vi "Timer_Start.vi"(8 "error in (no error)":errorcluster caption="错误输入（无错误）", 11 "Timer 输入":refnum<class "Timer.lvclass">) -> (0 "error out":errorcluster caption="错误输出", 3 "Timer 输出":refnum<class "Timer.lvclass">)   [LabVIEW 2019, in "Timer.lvclass"]
uses:
  Timer.lvclass
  Timer_Core.vi
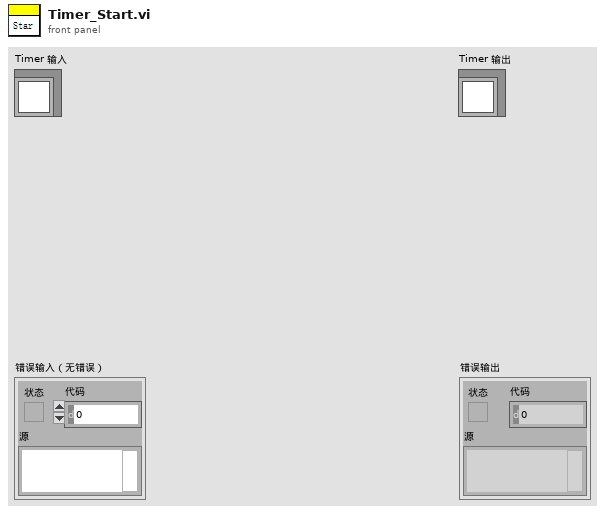
[diagram p1: front panel]
types:
  T1 = typedef "Timer.lvclass/Attribute.ctl" = cluster{"计时？":bool, "计时 (ms)":u32, "停止通知":refnum<notifier>}
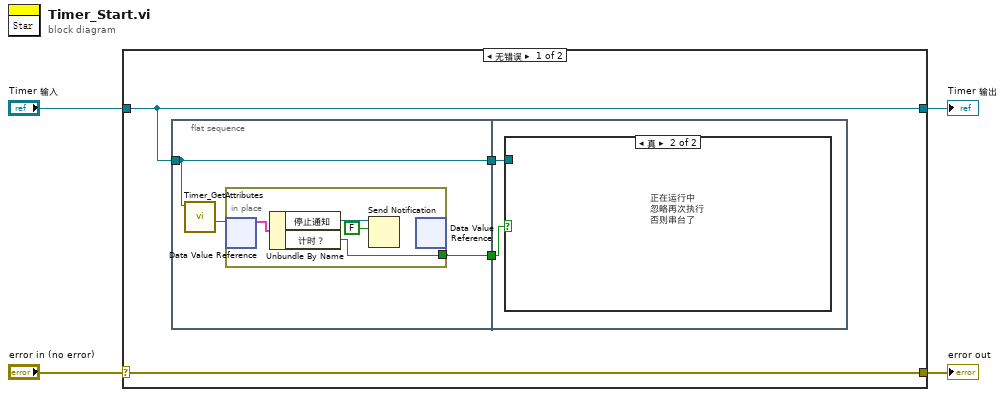
[diagram p0: block diagram]
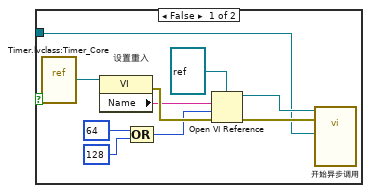
[diagram p2: hidden frame]
diagram:
  n1 = case shown="无错误" "error in (no error)" {
    selector: "error in (no error)" -> [w8 w29]
    tunnel: [w8 w29] -> w3
    tunnel: [w7 w28] -> w1
    tunnel: "Timer 输入" -> [w7 w28]
    frame No Error {
      n2 = flat-sequence {
        tunnel: w7 -> [w10]
        tunnel: [w10] -> w6
        tunnel: [w9] -> w5
        tunnel: w6 -> [w17]
        tunnel: w5 -> [w16]
        frame #0 {
          n3 = call "Timer_GetAttributes.vi"("Timer 输入"=w10) -> ("数据值引用"=w11:refnum<data-value>)  [unwired: 7 in, 3 out]
          n4 = in-place {
            in-place-border: [w12] -> w9
            n5 = in-place-dvr #1(w11) -> (w15:T1)  [unwired: 1 out]
            n6 = Unbundle By Name(w15) -> ("停止通知"=w14:refnum<notifier>, "计时？"=w12:bool)
            n7 = Send Notification(notification=FALSE ("通知"), notifier=w14) -> ()  [unwired: 1 in, 2 out]
            n8 = in-place-dvr #1() -> ()  [unwired: 1 in, 2 out]
          }
        }
        frame #1 {
          n9 = case shown="真" w16 {
            tunnel: w17 -> [w18 _]
            frame False {
              # "设置重入"
              n10 = vi-ref "Timer.lvclass:Timer_Core.vi"() -> (w22:refnum<vi>)
              n11 = property class="VI"(reference=w22) -> (error out=w25:errorcluster, "Name"=w23:string)  [unwired: 1 in, 1 out]
              n12 = Compound Arithmetic op=OR(64 ("options"), 128 ("options")) -> (w24:i32)
              n13 = Open VI Reference(type specifier VI Refnum (for type only)=refnum<vi> refnum ("类型说明符VI引用句柄（仅用于类型）"), vi path=w23, options=w24, error in (no error)=w25) -> (vi reference=w26:refnum<vi>, error out=w27:errorcluster)  [unwired: 2 in]
              n14 = call-by-ref "开始异步调用"(reference=w26, error in=w27, "Timer 输入"=w18) -> ()  [unwired: 9 in, 4 out]
            }
            frame True {
              # "正在运行中\n忽略再次执行\n否则串台了"
            }
          }
        }
      }
    }
    frame Error {
    }
  }
  "error out" <- w3
  "Timer 输出" <- w1
